vi "File_Torque.vi"() -> ()   [LabVIEW 2018]
panel:
  out "File_Torque (mNm)":dbl format="%.1f"
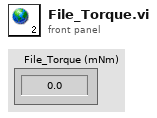
[diagram p1: front panel]
diagram:
